vi "Drive_Teleop.vi"(0 "Joystick_Out":T1, 2 "Visited_Disabled":bool) -> ()   [LabVIEW 2018]
uses:
  Utility_VIs/Joystick_Controls.ctl
  Subsytems/Drive/Drive_Notifier.ctl
  Subsytems/Drive/Drive_Control_Type.ctl
  Global_Variables/Drive_Globals.vi
  Global_Variables/Climb_Globals.vi
  Global_Variables/Sensor_Values.vi
  Global_Variables/Elevator_Globals.vi
  <vilib>/Rock Robotics/WPI/ThirdParty/Phoenix-LabVIEW/Motor Controller/Controls/CTRE_Phoenix_MotorControl_ControlMode.ctl
panel:
  out "Climb _Advance Drive":bool
  in  "Multiplier":dbl=1.0
  in  "Squared":bool=TRUE
  in  "Output Lower Limit":dbl=0.095
  in  "Band":dbl=0.1
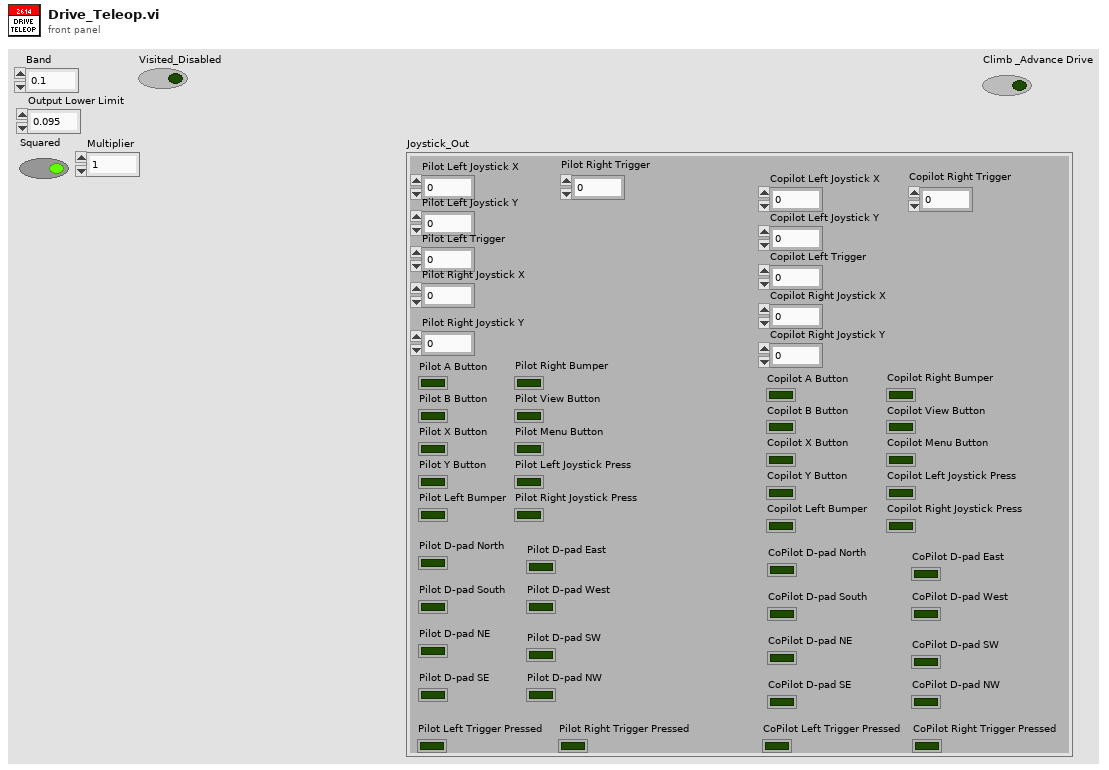
[diagram p1: front panel]
types:
  T1 = typedef "Joystick_Controls.ctl" = cluster{"Pilot Left Joystick X":dbl, "Pilot Left Joystick Y":dbl, "Pilot A Button":bool, "Pilot B Button":bool, "Pilot X Button":bool, "Pilot Y Button":bool, "Pilot Left Bumper":bool, "Pilot Right Bumper":bool, "Pilot View Button":bool, "Pilot Menu Button":bool, "Pilot Left Joystick Press":bool, "Pilot Right Joystick Press":bool, "Pilot Left Trigger":dbl, "Pilot Right Joystick X":dbl, "Pilot Right Joystick Y":dbl, "Pilot Right Trigger":dbl, "Copilot Left Joystick X":dbl, "Copilot Left Joystick Y":dbl, "Copilot A Button":bool, "Copilot B Button":bool, "Copilot X Button":bool, "Copilot Y Button":bool, "Copilot Left Bumper":bool, "Copilot Right Bumper":bool, "Copilot View Button":bool, "Copilot Menu Button":bool, "Copilot Left Joystick Press":bool, "Copilot Right Joystick Press":bool, "Copilot Left Trigger":dbl, "Copilot Right Joystick X":dbl, "Copilot Right Joystick Y":dbl, "Copilot Right Trigger":dbl, "Pilot D-pad North":bool, "Pilot D-pad South":bool, "Pilot D-pad East":bool, "Pilot D-pad West":bool, "Pilot D-pad NE ":bool, "Pilot D-pad SE":bool, "Pilot D-pad SW":bool, "Pilot D-pad NW":bool, "CoPilot D-pad North":bool, "CoPilot D-pad South":bool, "CoPilot D-pad East":bool, "CoPilot D-pad West":bool, "CoPilot D-pad NE":bool, "CoPilot D-pad SE":bool, "CoPilot D-pad SW":bool, "CoPilot D-pad NW":bool, "Pilot Left Trigger Pressed":bool, "Pilot Right Trigger Pressed":bool, "CoPilot Left Trigger Pressed":bool, "CoPilot Right Trigger Pressed":bool}
  T2 = typedef "Drive_Notifier.ctl" = cluster{"Drive Control List":T3, "Front/Back":dbl, "Left/Right":dbl, "Turn":dbl, "Test_Joy_Y":dbl, "Test_Joy_X":dbl, "Set Wheel Encoder Positions":bool, "Robotcentric":bool, "Reset Gyro":bool, "Rotate Front Right":bool, "Rotate Front Left":bool, "Rotate Back Right":bool, "Rotate Back Left":bool, "Write_Encoder_Positions":bool, "Climb_Advance":bool, "Parameter_One":dbl, "Parameter_Two":dbl, "Parameter_Three":dbl, "Parameter_Four":dbl, "Drive_Notifier":refnum<notifier>, "Step":i32, "Climb_Reverse":bool, "Auto_Target":bool}
  T3 = typedef "Drive_Control_Type.ctl" = enum16{"No_Op", "Write_FL_Position", "Write_FR_Position", "Write_BL_Position", "Write_BR_Position", "Set_Encoder_Positions", "Fieldcentric_PercentVBus", "Fieldcentric", "Robotcentric", "Reset_Gyro", "FR_Wheel", "FL_Wheel", "BR_Wheel", "BL_Wheel", "Drive_Onto_Platform", "Manual_Wheel_Control", "Distance", "Turn_To_Heading", "Turn_To_Target", "Drive_To_Target", "Zero", "Auto_Target", "Drive_Over_Platform", "Heading_Lock", "Time"}
  T4 = typedef "CTRE_Phoenix_MotorControl_ControlMode.ctl" = u16
  T5 = typedef "WPI_MotorControlDeviceRef.ctl" = cluster{"DeviceStatus":errorcluster, "Type":T6, "PWM":cluster{"PWM Channel":T7, "DeadBand":T8}, "CAN":cluster{"Device Number":u8, "SetOutput VI Ref":variant, "GetOutput VI Ref":variant, "Enable VI Ref":variant, "Disable VI Ref":variant, "Data":variant}, "Invert":bool, "DIO PWM":cluster{"PWM \"Enable\" Channel":T7, "DIOChannel":T9, "PWM Rate":dbl}}
  T6 = typedef "WPI_MotorControlType.ctl" = enum16{"PWM", "CAN", "DIO PWM"}
  T7 = typedef "FPGA_DIOPWMChannel.ctl" = enum8{"PWM 0", "PWM 1", "PWM 2", "PWM 3", "PWM 4", "PWM 5", "PWM 6", "PWM 7", "PWM 8", "PWM 9", "PWM MXP 0", "PWM MXP 1", "PWM MXP 2", "PWM MXP 3", "PWM MXP 4", "PWM MXP 5", "PWM MXP 6", "PWM MXP 7", "PWM MXP 8", "PWM MXP 9", "Invalid"}
  T8 = typedef "WPI_PWMDeadband.ctl" = cluster{"Name":string, "maxPositivePwm":i32, "minPositivePwm":i32, "centerPwm":i32, "maxNegativePwm":i32, "minNegativePwm":i32, "angularRange":u16}
  T9 = typedef "FPGA_DIOChannel.ctl" = enum8{"DIO 0", "DIO 1", "DIO 2", "DIO 3", "DIO 4", "DIO 5", "DIO 6", "DIO 7", "DIO 8", "DIO 9", "DIO MXP 0", "DIO MXP 1", "DIO MXP 2", "DIO MXP 3", "DIO MXP 4", "DIO MXP 5", "DIO MXP 6", "DIO MXP 7", "DIO MXP 8", "DIO MXP 9", "DIO MXP 10", "DIO MXP 11", "DIO MXP 12", "DIO MXP 13", "DIO MXP 14", "DIO MXP 15", "SPI Port CS1", "SPI Port CS2", "SPI Port CS3", "SPI Port MISO", "SPI Port MOSI", "Invalid"}
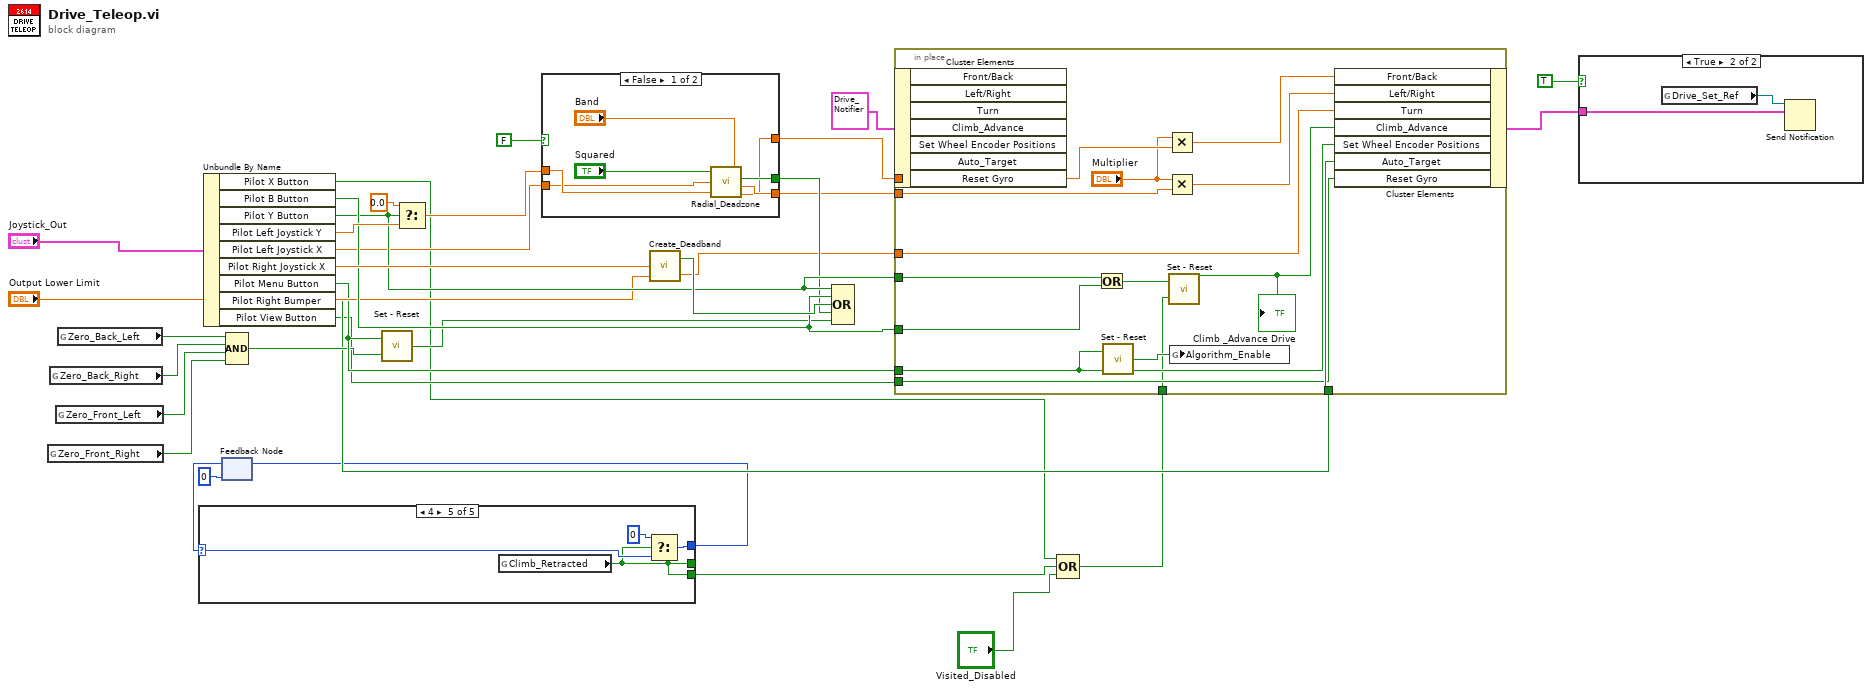
[diagram p0: block diagram]
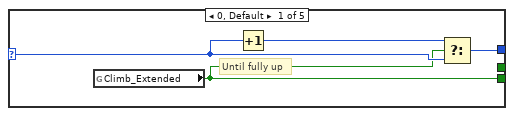
[diagram p2: hidden frame]
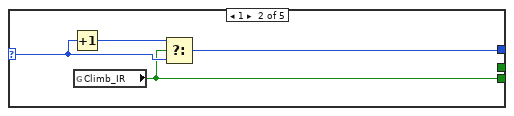
[diagram p3: hidden frame]
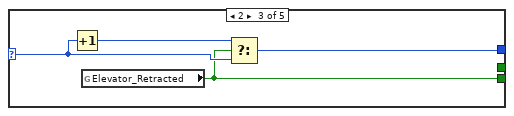
[diagram p4: hidden frame]
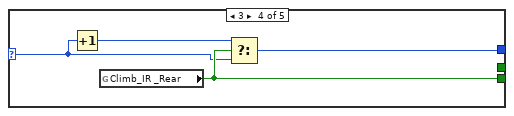
[diagram p5: hidden frame]
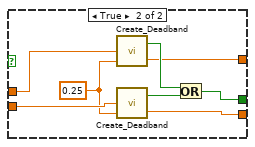
[diagram p6: hidden frame]
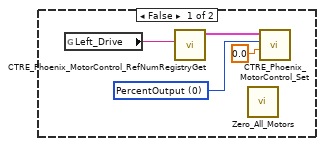
[diagram p7: hidden frame]
diagram:
  n1 = global read "Drive_Globals.vi" "Zero_Front_Right"() -> (w17:bool)
  n2 = global read "Drive_Globals.vi" "Zero_Back_Right"() -> (w15:bool)
  n3 = global read "Drive_Globals.vi" "Zero_Front_Left"() -> (w16:bool)
  n4 = global read "Drive_Globals.vi" "Zero_Back_Left"() -> (w14:bool)
  n5 = Unbundle By Name("Joystick_Out") -> ("Pilot X Button"=w2:bool, "Pilot B Button"=w27:bool, "Pilot Y Button"=w26:bool, "Pilot Left Joystick Y"=w29:dbl, "Pilot Left Joystick X"=w23:dbl, "Pilot Right Joystick X"=w31:dbl, "Pilot Menu Button"=w19:bool, "Pilot Right Bumper"=w10:bool, "Pilot View Button"=w8:bool)
  n6 = feedback #1(0) -> (w6:i32)
  n7 = case shown="4" w6 {
    selector: w6 -> [w37 w40 w44 w48 w53]
    tunnel: [w36 w42 w45 w50 w54] -> w5
    tunnel: [w35 w39 w43 w49 w51] -> w3
    tunnel: [_ _ _ _ w51] -> _
    frame 0, Default {
      # "Until fully up"
      n8 = global read "Climb_Globals.vi" "Climb_Extended"() -> (w35:bool)
      n9 = Increment(x=w37) -> (x+1=w38:i32)
      n10 = Select(t=w38, s=w35, f=w37) -> (s? t:f=w36:i32)
    }
    frame 1 {
      n11 = Increment(x=w40) -> (x+1=w41:i32)
      n12 = global read "Sensor_Values.vi" "Climb_IR"() -> (w39:bool)
      n13 = Select(t=w41, s=w39, f=w40) -> (s? t:f=w42:i32)
    }
    frame 2 {
      n14 = Increment(x=w44) -> (x+1=w46:i32)
      n15 = global read "Elevator_Globals.vi" "Elevator_Retracted"() -> (w43:bool)
      n16 = Select(t=w46, s=w43, f=w44) -> (s? t:f=w45:i32)
    }
    frame 3 {
      n17 = Increment(x=w48) -> (x+1=w47:i32)
      n18 = global read "Sensor_Values.vi" "Climb_IR _Rear"() -> (w49:bool)
      n19 = Select(t=w47, s=w49, f=w48) -> (s? t:f=w50:i32)
    }
    frame 4 {
      n20 = global read "Climb_Globals.vi" "Climb_Retracted"() -> (w51:bool)
      n21 = Select(t=0, s=w51, f=w53) -> (s? t:f=w54:i32)
    }
  }
  n22 = feedback-in #1(w5) -> ()
  n23 = Compound Arithmetic op=AND(w14, w15, w16, w17) -> (w13:bool)
  n24 = call "Set - Reset.vi"("Reset"=w13, "Set"=w19) -> ("Output"=w18:bool)
  n25 = Select(t=0.0, s=w26, f=w29) -> (s? t:f=w24:dbl)
  n26 = case shown="False" FALSE {
    tunnel: [w61 w69] -> w25
    tunnel: w24 -> [w60 w63]
    tunnel: w23 -> [w59 w64]
    tunnel: [w58 w66] -> w22
    tunnel: [w57 w65] -> w21
    frame False {
      n27 = call "Radial_Deadzone.vi"("Squared"="Squared", "X"=w59, "Y"=w60, "Band"="Band") -> ("Not_Zero"=w61:bool, "X_Out"=w58:dbl, "Y_Out"=w57:dbl)
    }
    frame True {
      w62 = 0.25
      n28 = call "Create_Deadband.vi"("Output Lower Limit"=w62, "Input"=w63) -> ("Output"=w65:dbl, "Not Zero?"=w67:bool)  [unwired: 1 in]
      n29 = call "Create_Deadband.vi"("Output Lower Limit"=w62, "Input"=w64) -> ("Output"=w66:dbl, "Not Zero?"=w68:bool)  [unwired: 1 in]
      n30 = Or(x=w67, y=w68) -> (x .or. y?=w69:bool)
    }
  }
  n31 = call "Create_Deadband.vi"("Output Lower Limit"="Output Lower Limit", "Input"=w31) -> ("Output"=w9:dbl, "Not Zero?"=w28:bool)  [unwired: 1 in]
  n32 = Compound Arithmetic op=OR(w26, w27, w28, w25, w18) -> ()  [unwired: 1 out]
  n33 = Compound Arithmetic op=OR(w2, w3, "Visited_Disabled") -> (w4:bool)
  n34 = in-place {
    in-place-border: w9 -> [w84]
    in-place-border: w26 -> [w83]
    in-place-border: w27 -> [w82]
    in-place-border: w22 -> [w78]
    in-place-border: w21 -> [w79]
    in-place-border: w19 -> [w81]
    in-place-border: w10 -> [w74]
    in-place-border: w8 -> [w73]
    in-place-border: w4 -> [w70]
    n35 = in-place-cluster #2 ("Unbundle / Bundle Elements")(T2 {"Drive Control List"=enum."No_Op", "Front/Back"=0.0, "Left/Right"=0.0, "Turn"=0.0, "Test_Joy_Y"=0.0, "Test_Joy_X"=0.0, "Set Wheel Encoder Positions"=FALSE, "Robotcentric"=FALSE, "Reset Gyro"=FALSE, "Rotate Front Right"=FALSE, "Rotate Front Left"=FALSE, "Rotate Back Right"=FALSE, "Rotate Back Left"=FALSE, "Write_Encoder_Positions"=FALSE, "Climb_Advance"=FALSE, "Parameter_One"=0.0, "Parameter_Two"=0.0, "Parameter_Three"=0.0, "Parameter_Four"=0.0, "Drive_Notifier"=refnum, "Step"=0, "Climb_Reverse"=FALSE, "Auto_Target"=FALSE} ("Drive Notifier")) -> ()  [unwired: 7 out]
    n36 = Or(x=w83, y=w82) -> (x .or. y?=w71:bool)
    n37 = call "Set - Reset.vi"("Set"=w81) -> ("Output"=w80:bool)  [unwired: 1 in]
    n38 = Multiply(x="Multiplier", y=w79) -> (x*y=w77:dbl)
    n39 = Multiply(x="Multiplier", y=w78) -> (x*y=w76:dbl)
    n40 = call "Set - Reset.vi"("Reset"=w70, "Set"=w71) -> ("Output"=w72:bool)
    "Climb _Advance Drive" <- w72
    n41 = global write "Drive_Globals.vi" "Algorithm_Enable"(w80) -> ()
    n42 = in-place-cluster #2("Front/Back"=w77, "Left/Right"=w76, "Turn"=w84, "Climb_Advance"=w72, "Set Wheel Encoder Positions"=w81, "Auto_Target"=w74, "Reset Gyro"=w73) -> (w33:T2)
  }
  n43 = case shown="True" TRUE {
    tunnel: w33 -> [_ w90]
    frame False {
      w85 = T4 0 items=["PercentOutput"=0, "Position"=1, "Velocity"=2, "Current"=3, "Follower"=5, "MotionProfile"=6, "MotionMagic"=7, "MotionProfileArc"=10, "Disabled"=15] ("Control Mode")
      n44 = global read "Climb_Globals.vi" "Left_Drive"() -> (w88:string)
      n45 = call <vilib>:"CTRE_Phoenix_MotorControl_RefNumRegistryGet.vi"("refnum name"=w88) -> ("PhoenixMotorControlDevRef"=w87:T5)  [unwired: 9 in, 1 out]
      n46 = call "Zero_All_Motors.vi"() -> ()  [unwired: 12 in]
      n47 = call <vilib>:"CTRE_Phoenix_MotorControl_Set.vi"("Output"=0.0, "Control Mode"=w85, "PhoenixMotorControlDevRef"=w87) -> ()  [unwired: 7 in, 2 out]
    }
    frame True {
      n48 = global read "Drive_Globals.vi" "Drive_Set_Ref"() -> (w89:refnum<notifier>)
      n49 = Send Notification(notification=w90, notifier=w89) -> ()  [unwired: 1 in, 2 out]
    }
  }
